vi "Interp_waveform_galvos_DB.vi"(2 "autospiral":bool, 3 "numpoints":dbl, 4 "cycles in spiral":dbl, 5 "XY Volt":T1) -> (0 "Y-Wave":dbl[](array[numeric]), 1 "X-Wave":dbl[](array[numeric]))   [LabVIEW 2013]
uses:
  <vilib>/Analysis/Matrix/Datatypes/RealMatrix.ctl
  <vilib>/Analysis/Matrix/Numeric/Conversions/Matrix To Array - RM.vi
  <vilib>/Analysis/Matrix/NI_Matrix.lvlib
  <vilib>/measure/NI_MABase.lvlib
panel:
  out "Waveform Chart":waveform(dbl)(graph)
  out "X-Y Graph 3":T2(graph)
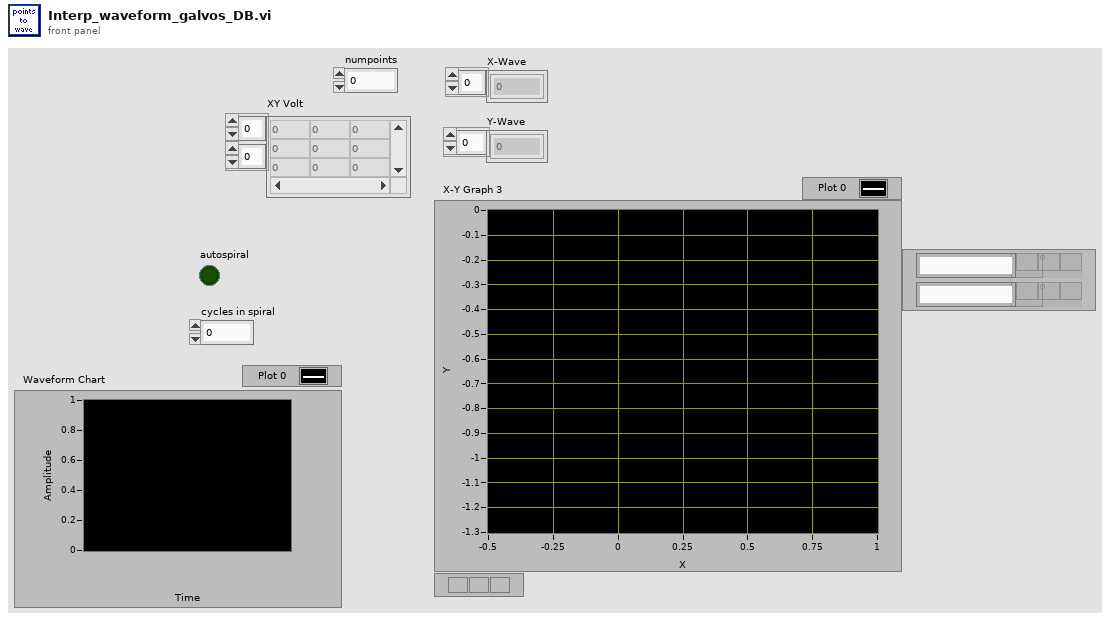
[diagram p1: front panel]
types:
  T1 = typedef "NI_Matrix.lvlib/RealMatrix.ctl" = dbl[][]
  T2 = cluster{"X-WaveArray":dbl[], "Y-WaveArray":dbl[]}[]
  T3 = cluster{"Real 2D Array":dbl[], "Real 2D Array":dbl[]}
  T4 = cluster{"Real 2D Array":dbl[], "Real 2D Array":dbl[]}[]
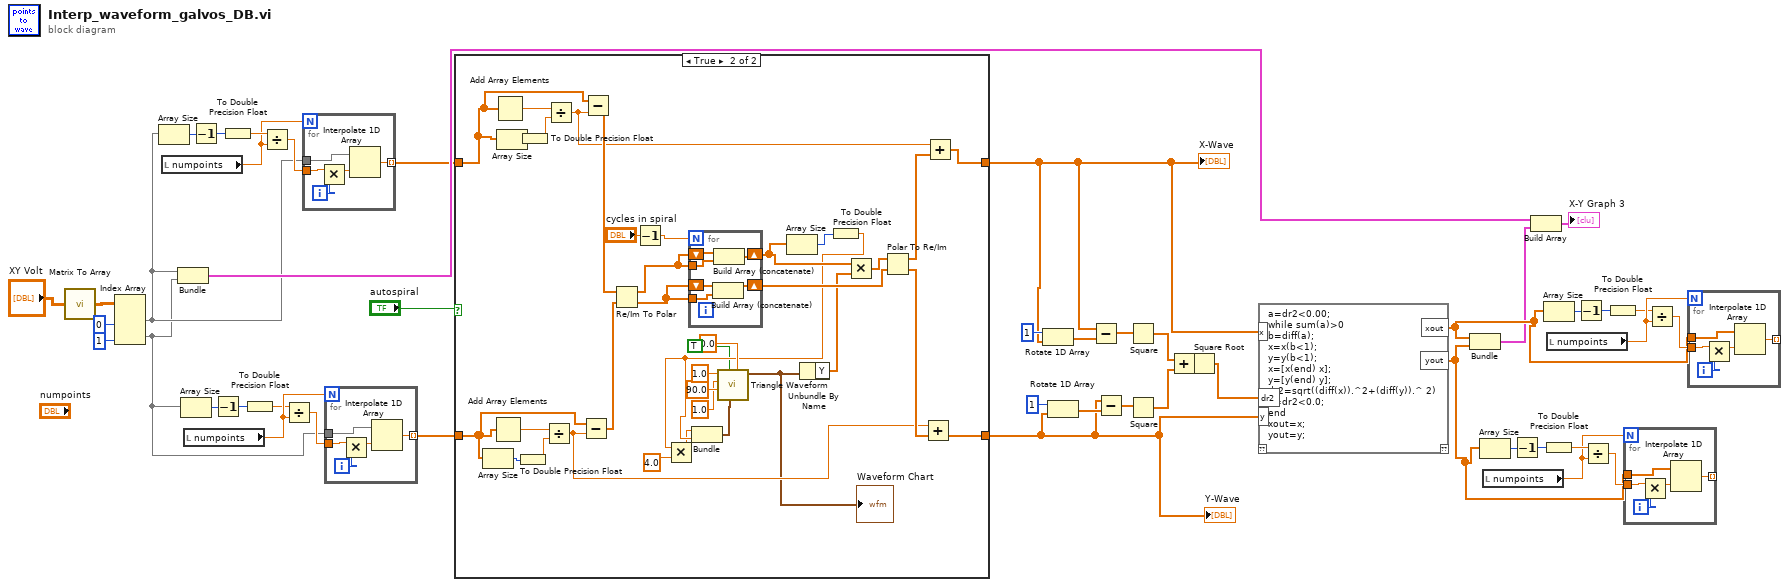
[diagram p0: block diagram]
diagram:
  n1 = call-poly <vilib>:"Matrix To Array.vi"("Real Matrix"="XY Volt") -> ("Real 2D Array"=w12:dbl[][])
  n2 = Index Array(array=w12, index (col) #1=0 ("disabled index (col)"), index (col) #2=1 ("index (col)")) -> (element #1=w10:dbl[], element #2=w8:dbl[])  [unwired: 2 in]
  n3 = Array Size(array=w10) -> (size(s)=w34:i32)
  n4 = local read "numpoints"() -> (w7:dbl)
  n5 = Bundle("Real 2D Array"=w10, "Real 2D Array"=w8) -> (w37:T3)  [unwired: 1 in]
  n6 = Array Size(array=w8) -> (size(s)=w26:i32)
  n7 = local read "numpoints"() -> (w30:dbl)
  n8 = Decrement(x=w34) -> (x-1=w33:i32)
  n9 = Decrement(x=w26) -> (x-1=w27:i32)
  n10 = To Double Precision Float(number=w33) -> (double precision float=w32:dbl)
  n11 = To Double Precision Float(number=w27) -> (double precision float=w28:dbl)
  n12 = Divide(x=w32, y=w7) -> (x/y=w31:dbl)
  n13 = Divide(x=w28, y=w30) -> (x/y=w29:dbl)
  n14 = for {
    N: w7 -> [_]
    tunnel: w10 -> [w51]
    tunnel: w31 -> [w50]
    tunnel: [w49] -> w6 mode=indexing
    i -> [w47]
    n15 = Multiply(x=w50, y=w47) -> (x*y=w48:dbl)
    n16 = Interpolate 1D Array(1:w48, 2:w51) -> (0:w49:dbl)
  }
  n17 = for {
    N: w30 -> [_]
    tunnel: w8 -> [w56]
    tunnel: w29 -> [w55]
    tunnel: [w54] -> w5 mode=indexing
    i -> [w52]
    n18 = Multiply(x=w55, y=w52) -> (x*y=w53:dbl)
    n19 = Interpolate 1D Array(1:w53, 2:w56) -> (0:w54:dbl)
  }
  n20 = case shown="True" "autospiral" {
    tunnel: w6 -> [w58 w87]
    tunnel: [w58 w66] -> w1
    tunnel: w5 -> [w57 w86]
    tunnel: [w57 w65] -> w2
    frame False {
    }
    frame True {
      n21 = Array Size(array=w86) -> (size(s)=w89:i32)
      n22 = Add Array Elements(numeric array=w86) -> (sum=w88:dbl)
      n23 = Add Array Elements(numeric array=w87) -> (sum=w93:dbl)
      n24 = Array Size(array=w87) -> (size(s)=w92:i32)
      n25 = To Double Precision Float(number=w89) -> (double precision float=w90:dbl)
      n26 = To Double Precision Float(number=w92) -> (double precision float=w91:dbl)
      n27 = Divide(x=w88, y=w90) -> (x/y=w64:dbl)
      n28 = Divide(x=w93, y=w91) -> (x/y=w67:dbl)
      n29 = Subtract(x=w86, y=w64) -> (x-y=w84:dbl[])
      n30 = Subtract(x=w87, y=w67) -> (x-y=w85:dbl[])
      n31 = Re/Im To Polar(2:w84, 3:w85) -> (0:w80:dbl[], 1:w81:dbl[])
      n32 = Decrement(x="cycles in spiral") -> (x-1=w82:dbl)
      n33 = for {
        N: w82 -> [_]
        shift-right: [w97] -> w72
        shift-left: w81 -> [w98]
        tunnel: w81 -> [w99]
        shift-right: [w94] -> w70
        shift-left: w80 -> [w96]
        tunnel: w80 -> [w95]
        n34 = Build Array (concatenate)(w96, w95) -> (w94:dbl[])
        n35 = Build Array (concatenate)(w98, w99) -> (w97:dbl[])
      }
      n36 = Array Size(array=w72) -> (size(s)=w78:i32)
      n37 = To Double Precision Float(number=w78) -> (double precision float=w61:dbl)
      n38 = Multiply(x=w61, y=4.0) -> (x*y=w60:dbl)
      n39 = Bundle(w60, w61) -> (w76:cluster{dbl, dbl})  [unwired: 1 in]
      n40 = call <vilib>:"Triangle Waveform.vi"("offset"=0.0, "sampling info"=w76, "reset signal"=TRUE, "phase"=90.0, "amplitude"=1.0, "frequency"=1.0) -> ("signal out"=w62:waveform(dbl))  [unwired: 4 in, 1 out]
      "Waveform Chart" <- w62
      n41 = Unbundle By Name(w62) -> ("Y"=w63:dbl[])
      n42 = Multiply(x=w72, y=w63) -> (x*y=w71:dbl[])
      n43 = Polar To Re/Im(2:w70, 3:w71) -> (0:w69:dbl[], 1:w68:dbl[])
      n44 = Add(x=w64, y=w69) -> (x+y=w65:dbl[])
      n45 = Add(x=w67, y=w68) -> (x+y=w66:dbl[])
    }
  }
  "X-Wave" <- w1
  "Y-Wave" <- w2
  n46 = Rotate 1D Array(1:w1, 2:1 ("n")) -> (0:w45:dbl[])
  n47 = Rotate 1D Array(1:w2, 2:1 ("n")) -> (0:w44:dbl[])
  n48 = Subtract(x=w1, y=w45) -> (x-y=w42:dbl[])
  n49 = Subtract(x=w2, y=w44) -> (x-y=w41:dbl[])
  n50 = Square(x=w42) -> (x^2=w40:dbl[])
  n51 = Square(x=w41) -> (x^2=w39:dbl[])
  n52 = Add(x=w40, y=w39) -> (x+y=w38:dbl[])
  n53 = Square Root(x=w38) -> (sqrt(x)=w35:dbl[])
  n54 = script code="a=dr2<0.00;\nwhile sum(a)>0\nb=diff(a);\nx=x(b<1);\ny=y(b<1);\nx=[x(end) x];\ny=[y(end) y];\ndr2=sqrt((diff(x)).^2+(diff(y)).^ 2)\na=dr2<0.0;\nend\nxout=x;\nyout=y;"("dr2"=w35, "x"=w1, "y"=w2) -> ("xout"=w20:dbl[], "yout"=w14:dbl[])  [unwired: 1 in, 1 out]
  n55 = Bundle(w20, w14) -> (w3:cluster{dbl[], dbl[]})  [unwired: 1 in]
  n56 = Array Size(array=w14) -> (size(s)=w19:i32)
  n57 = local read "numpoints"() -> (w15:dbl)
  n58 = Decrement(x=w19) -> (x-1=w18:i32)
  n59 = Build Array(w37, w3) -> (→"X-Y Graph 3":T4)
  n60 = Array Size(array=w20) -> (size(s)=w21:i32)
  n61 = To Double Precision Float(number=w18) -> (double precision float=w17:dbl)
  n62 = local read "numpoints"() -> (w25:dbl)
  n63 = Decrement(x=w21) -> (x-1=w22:i32)
  n64 = Divide(x=w17, y=w15) -> (x/y=w16:dbl)
  n65 = To Double Precision Float(number=w22) -> (double precision float=w23:dbl)
  n66 = for {
    N: w15 -> [_]
    tunnel: w14 -> [w104]
    tunnel: w16 -> [w103]
    tunnel: [w102] -> _ mode=indexing
    i -> [w100]
    n67 = Multiply(x=w103, y=w100) -> (x*y=w101:dbl)
    n68 = Interpolate 1D Array(1:w101, 2:w104) -> (0:w102:dbl)
  }
  n69 = Divide(x=w23, y=w25) -> (x/y=w24:dbl)
  n70 = for {
    N: w25 -> [_]
    tunnel: w20 -> [w109]
    tunnel: w24 -> [w108]
    tunnel: [w107] -> _ mode=indexing
    i -> [w105]
    n71 = Multiply(x=w108, y=w105) -> (x*y=w106:dbl)
    n72 = Interpolate 1D Array(1:w106, 2:w109) -> (0:w107:dbl)
  }
